vi "Gen - Check for Repeating User Event.vi"(11 "Time":u32) -> (3 "Repeat?":bool)   [LabVIEW 2020]
doc: "This VI use to check for a repeated event. If a new event occured within 500 ms, that event is ignored.\n\nIn some cases, there is a case that handle task more than 500 ms. To avoid the software lagging on user event case, this VI will check a time between two event. A new event occurred within 500 ms is ignored."
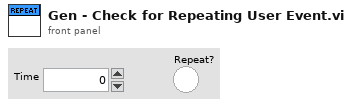
[diagram p1: front panel]
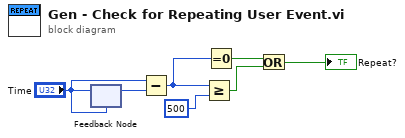
[diagram p0: block diagram]
diagram:
  n1 = feedback #1("Time") -> (w7:u32)
  n2 = feedback-in #1("Time") -> ()
  n3 = Subtract(x="Time", y=w7) -> (x-y=w4:u32)
  n4 = Greater Or Equal?(x=w4, y=u32 500) -> (x >= y?=w2:bool)
  n5 = Equal To 0?(x=w4) -> (x = 0?=w3:bool)
  n6 = Or(x=w3, y=w2) -> (x .or. y?=→"Repeat?":bool)
